vi "Log Data.vi"(0 "Log Data":bool[](array[boolean]), 1 "Log AKLH":bool[](array[boolean]), 2 "Data Log Dirs":path[](array[path]), 3 "AKLH Today Dirs":path[](array[path]), 4 "Record Time (sec)":dbl, 5 "Target Speed":string, 6 "Profile":string[][](array[string]), 7 "Current Step":i32=2, 8 "Pump Data":T3={"Voltages"=[0.015201568603515625, 0.00335693359375, 0.003021240234375, 0.12260055541992188, 0.06085968017578125, 0.052234649658203125], "PumpCurrent"=[0.015201568603515625, 0.00335693359375, 0.003021240234375, 0.12260055541992188, 0.06085968017578125, 0.052234649658203125], "Speed"=[0.0, 0.0, 0.0, 0.0, 0.0, 0.0], "ControllerCurrent"=[0.015201568603515625, 0.00335693359375, 0.003021240234375, 0.12260055541992188, 0.06085968017578125, 0.052234649658203125], "Pressure"=[0.015201568603515625, 0.00335693359375, 0.003021240234375, 0.12260055541992188, 0.06085968017578125, 0.052234649658203125], "Flow"=[0.0, 0.0, 0.0, 0.125, 0.0625, 0.0625], "Elapsed Time (Display)"=[7.1, 7.1, 7.1, 458133.45, 458138.85000000003, 458126.75], "Avg Pressure"=0.0, "Avg Speed"=0.0, "Elapsed Time"=[4074.9003000000002, 4074.9003000000002, 4074.9003000000002, 4074.9003000000002, 4074.9003000000002, 4074.9003000000002]} {"Elapsed Time" format="%<%H:%M:%S>t"; "Elapsed Time (Display)" format="%<%H:%M:%S>t"; "Speed" format="%#_4f"; "ControllerCurrent" format="%#.1g"; "Pressure" format="%#.0f"; "Flow" format="%#.0f"; "PumpCurrent" format="%#.1g"; "Voltages" format="%#.0f"}, 9 "Tank CMDs":T1, 10 "Tank Data":T2 {"PS Actual (V):" format="%.2f"; "Temp1" format="%#_2g"; "Temp2" format="%#_2g"}, 11 "AKLH Filename":string, 13 "3 Pump Tank":bool) -> ()   [LabVIEW 2018]
uses:
  Controls/Pump Data.ctl
  Controls/Tank Data.ctl
  Controls/Tank CMDs.ctl
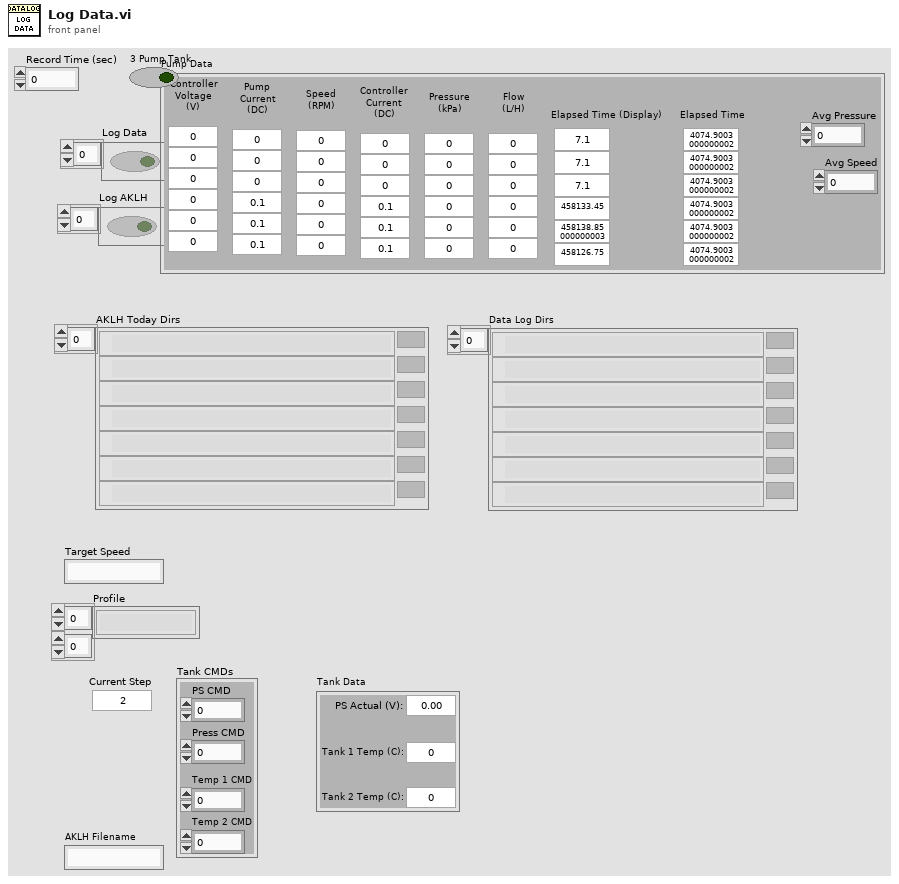
[diagram p1: front panel]
types:
  T1 = typedef "Tank CMDs.ctl" = cluster{"PS CMD":dbl, "Press CMD":dbl, "Temp 1 CMD":dbl, "Temp 2 CMD":dbl}
  T2 = typedef "Tank Data.ctl" = cluster{"PS Actual (V):":dbl, "Temp1":dbl, "Temp2":dbl}
  T3 = typedef "Pump Data.ctl" = cluster{"Voltages":dbl[], "PumpCurrent":dbl[], "Speed":dbl[], "ControllerCurrent":dbl[], "Pressure":dbl[], "Flow":dbl[], "Elapsed Time (Display)":dbl[], "Avg Pressure":dbl, "Avg Speed":dbl, "Elapsed Time":dbl[]}
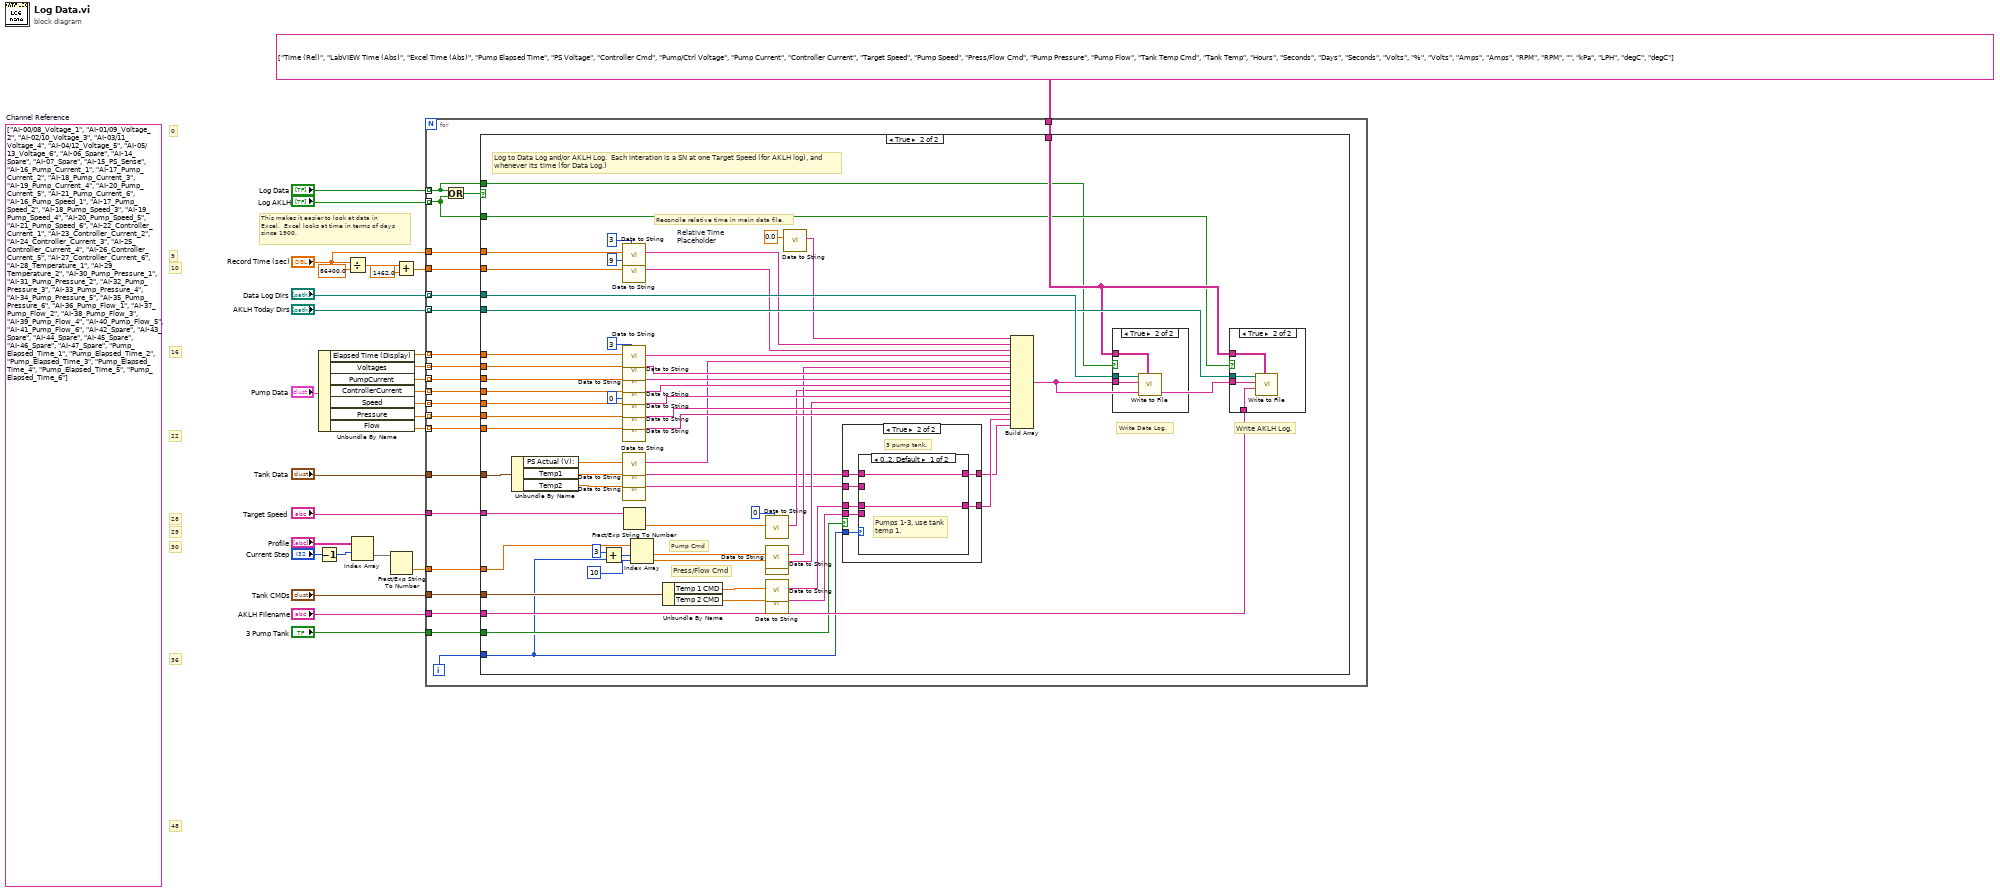
[diagram p0: block diagram]
diagram:
  (unwired) string[] ["AI-00/08_Voltage_1", "AI-01/09_Voltage_2", "AI-02/10_Voltage_3", "AI-03/11_Voltage_4", "AI-04/12_Voltage_5", "AI-05/13_Voltage_6", "AI-06_Spare", "AI-14_Spare", "AI-07_Spare", "AI-15_PS_Sense", "AI-16_Pump_Current_1", "AI-17_Pump_Current_2", "AI-18_Pump_Current_3", "AI-19_Pump_Current_4", "AI-20_Pump_Current_5", "AI-21_Pump_Current_6", "AI-16_Pump_Speed_1", "AI-17_Pump_Speed_2", "AI-18_Pump_Speed_3", "AI-19_Pump_Speed_4", "AI-20_Pump_Speed_5", "AI-21_Pump_Speed_6", "AI-22_Controller_Current_1", "AI-23_Controller_Current_2", "AI-24_Controller_Current_3", "AI-25_Controller_Current_4", "AI-26_Controller_Current_5", "AI-27_Controller_Current_6", "AI-28_Temperature_1", "AI-29_Temperature_2", "AI-30_Pump_Pressure_1", "AI-31_Pump_Pressure_2", "AI-32_Pump_Pressure_3", "AI-33_Pump_Pressure_4", "AI-34_Pump_Pressure_5", "AI-35_Pump_Pressure_6", "AI-36_Pump_Flow_1", "AI-37_Pump_Flow_2", "AI-38_Pump_Flow_3", "AI-39_Pump_Flow_4", "AI-40_Pump_Flow_5", "AI-41_Pump_Flow_6", "AI-42_Spare", "AI-43_Spare", "AI-44_Spare", "AI-45_Spare", "AI-46_Spare", "AI-47_Spare", "Pump_Elapsed_Time_1", "Pump_Elapsed_Time_2", "Pump_Elapsed_Time_3", "Pump_Elapsed_Time_4", "Pump_Elapsed_Time_5", "Pump_Elapsed_Time_6"]  # Channel Reference
  # "This makes it easier to look at data in\nExcel.  Excel looks at time in terms of days\nsince 1900."
  # "36"
  # "30"
  # "29"
  # "28"
  # "22"
  # "16"
  # "10"
  # "9"
  # "0"
  # "48"
  n1 = Decrement(x="Current Step") -> (x-1=w19:i32)
  n2 = Unbundle By Name("Pump Data") -> ("Elapsed Time (Display)"=w15:dbl[], "Voltages"=w14:dbl[], "PumpCurrent"=w13:dbl[], "ControllerCurrent"=w12:dbl[], "Speed"=w11:dbl[], "Pressure"=w10:dbl[], "Flow"=w9:dbl[])
  n3 = Divide(x="Record Time (sec)", y=86400.0) -> (x/y=w5:dbl)
  n4 = Index Array(array="Profile", index (row)=w19) -> (element=w18:string[])  [unwired: 1 in]
  n5 = Fract/Exp String To Number(string=w18) -> (number=w17:dbl[])  [unwired: 3 in, 1 out]
  n6 = Add(x=w5, y=1462.0) -> (x+y=w2:dbl)
  n7 = for {
    tunnel: "Data Log Dirs" -> [w50] mode=indexing
    tunnel: "AKLH Today Dirs" -> [w49] mode=indexing
    tunnel: "Record Time (sec)" -> [w48]
    tunnel: "AKLH Filename" -> [w46]
    tunnel: "Target Speed" -> [w45]
    tunnel: "Tank CMDs" -> [w44]
    tunnel: string[][] [["Time (Rel)", "LabVIEW Time (Abs)", "Excel Time (Abs)", "Pump Elapsed Time", "PS Voltage", "Controller Cmd", "Pump/Ctrl Voltage", "Pump Current", "Controller Current", "Target Speed", "Pump Speed", "Press/Flow Cmd", "Pump Pressure", "Pump Flow", "Tank Temp Cmd", "Tank Temp"], ["Hours", "Seconds", "Days", "Seconds", "Volts", "%", "Volts", "Amps", "Amps", "RPM", "RPM", "", "kPa", "LPH", "degC", "degC"]] ("subarray") -> [w43]
    tunnel: "Log Data" -> [w41] mode=indexing
    tunnel: "Log AKLH" -> [w40] mode=indexing
    tunnel: w17 -> [w39]
    tunnel: w15 -> [w37] mode=indexing
    tunnel: w14 -> [w36] mode=indexing
    tunnel: w13 -> [w35] mode=indexing
    tunnel: w12 -> [w34] mode=indexing
    tunnel: w11 -> [w33] mode=indexing
    tunnel: w10 -> [w32] mode=indexing
    tunnel: w9 -> [w31] mode=indexing
    tunnel: "Tank Data" -> [w38]
    tunnel: w2 -> [w30]
    tunnel: "3 Pump Tank" -> [w29]
    i -> [w47]
    n8 = Or(x=w41, y=w40) -> (x .or. y?=w42:bool)
    n9 = case shown="True" w42 {
      tunnel: w50 -> [_ w108]
      tunnel: w49 -> [_ w107]
      tunnel: w48 -> [_ w96]
      tunnel: w41 -> [_ w102]
      tunnel: w47 -> [_ w53]
      tunnel: w46 -> [_ w104]
      tunnel: w45 -> [_ w62]
      tunnel: w44 -> [_ w109]
      tunnel: w43 -> [_ w106]
      tunnel: w40 -> [_ w103]
      tunnel: w39 -> [_ w101]
      tunnel: w38 -> [_ w100]
      tunnel: w37 -> [_ w91]
      tunnel: w36 -> [_ w85]
      tunnel: w35 -> [_ w83]
      tunnel: w34 -> [_ w81]
      tunnel: w33 -> [_ w79]
      tunnel: w32 -> [_ w76]
      tunnel: w31 -> [_ w74]
      tunnel: w30 -> [_ w94]
      tunnel: w29 -> [_ w58]
      frame False {
        # "Neither Data Log is ready to log, nor pump in spec."
      }
      frame True {
        w87 = 0.0  # Relative Time Placeholder
        # "Press/Flow Cmd"
        # "Pump Cmd"
        # "Reconcile relative time in main data file."
        # "Write AKLH Log."
        # "Write Data Log."
        # "Log to Data Log and/or AKLH Log.  Each interation is a SN at one Target Speed (for AKLH log), and\nwhenever its time (for Data Log.)"
        n10 = Unbundle By Name(w100) -> ("PS Actual (V):"=w72:dbl, "Temp1"=w70:dbl, "Temp2"=w69:dbl)
        n11 = Add(x=3, y=w53) -> (x+y=w98:i32)
        n12 = call "Data to String.vi"("Precision (2)"=i16 3, "Data"=w96) -> ("String Data"=w95:string)  [unwired: 9 in]
        n13 = call "Data to String.vi"("Precision (2)"=i16 9, "Data"=w94) -> ("String Data"=w93:string)  [unwired: 9 in]
        n14 = call "Data to String.vi"("Precision (2)"=i16 3, "Data"=w91) -> ("String Data"=w90:string)  [unwired: 9 in]
        n15 = call "Data to String.vi"("Data"=w85) -> ("String Data"=w84:string)  [unwired: 10 in]
        n16 = call "Data to String.vi"("Data"=w83) -> ("String Data"=w82:string)  [unwired: 10 in]
        n17 = call "Data to String.vi"("Data"=w81) -> ("String Data"=w80:string)  [unwired: 10 in]
        n18 = call "Data to String.vi"("Precision (2)"=i16 0, "Data"=w79) -> ("String Data"=w78:string)  [unwired: 9 in]
        n19 = call "Data to String.vi"("Data"=w76) -> ("String Data"=w75:string)  [unwired: 10 in]
        n20 = call "Data to String.vi"("Data"=w74) -> ("String Data"=w73:string)  [unwired: 10 in]
        n21 = call "Data to String.vi"("Data"=w72) -> ("String Data"=w71:string)  [unwired: 10 in]
        n22 = call "Data to String.vi"("Data"=w70) -> ("String Data"=w55:string)  [unwired: 10 in]
        n23 = call "Data to String.vi"("Data"=w69) -> ("String Data"=w52:string)  [unwired: 10 in]
        n24 = Fract/Exp String To Number(string=w62) -> (number=w61:dbl)  [unwired: 3 in, 1 out]
        n25 = Index Array(array=w101, index #1=w98, index #2=10 ("x")) -> (element #1=w68:dbl, element #2=w66:dbl)
        n26 = Unbundle By Name(w109) -> ("Temp 1 CMD"=w64:dbl, "Temp 2 CMD"=w63:dbl)
        n27 = call "Data to String.vi"("Precision (2)"=i16 0, "Data"=w61) -> ("String Data"=w59:string)  [unwired: 9 in]
        n28 = call "Data to String.vi"("Data"=w68) -> ("String Data"=w67:string)  [unwired: 10 in]
        n29 = call "Data to String.vi"("Data"=w66) -> ("String Data"=w65:string)  [unwired: 10 in]
        n30 = call "Data to String.vi"("Data"=w64) -> ("String Data"=w57:string)  [unwired: 10 in]
        n31 = call "Data to String.vi"("Data"=w63) -> ("String Data"=w51:string)  [unwired: 10 in]
        n32 = call "Data to String.vi"("Data"=w87) -> ("String Data"=w86:string)  [unwired: 10 in]
        n33 = case shown="True" w58 {
          tunnel: w57 -> [w111 w115]
          tunnel: [w111 w114] -> w56
          tunnel: [w110 w116] -> w54
          tunnel: w55 -> [w110 w117]
          tunnel: w53 -> [_ w118]
          tunnel: w52 -> [_ w113]
          tunnel: w51 -> [_ w112]
          frame False {
            # "Only one tank, so use\ntank temp 1."
            # "6 pump tank."
          }
          frame True {
            # "3 pump tank."
            n34 = case shown="0..2, Default" w118 {
              tunnel: [w120 w122] -> w116
              tunnel: w117 -> [w120 _]
              tunnel: [w119 w121] -> w114
              tunnel: w115 -> [w119 _]
              tunnel: w113 -> [_ w122]
              tunnel: w112 -> [_ w121]
              frame 0..2, Default {
                # "Pumps 1-3, use tank\ntemp 1."
              }
              frame 3..5 {
                # "Pumps 4-6, use tank\ntemp 2."
              }
            }
          }
        }
        n35 = Build Array(w86, w95, w93, w90, w71, w67, w84, w82, w80, w59, w78, w65, w75, w73, w56, w54) -> (w105:string[])
        n36 = case shown="True" w102 {
          tunnel: w108 -> [_ w129]
          tunnel: w106 -> [_ w128]
          tunnel: w105 -> [_ w127]
          frame False {
          }
          frame True {
            n37 = call "Write to File.vi"("Column Header"=w128, "Data"=w127, "Path"=w129) -> ()  [unwired: 9 in]
          }
        }
        n38 = case shown="True" w103 {
          tunnel: w107 -> [_ w126]
          tunnel: w106 -> [_ w125]
          tunnel: w105 -> [_ w124]
          tunnel: w104 -> [_ w123]
          frame False {
          }
          frame True {
            n39 = call "Write to File.vi"("Column Header"=w125, "Filename"=w123, "Data"=w124, "Path"=w126) -> ()  [unwired: 8 in]
          }
        }
      }
    }
  }
